vi "Complex Matrix Trace.vi"(0 "Input Matrix":T1) -> (1 "trace":cdb format="%.2f", 2 "error":i32)   [LabVIEW 2014, in "NI_AALPro.lvlib"]
doc: "Finds the <B>trace</B> of <B>Input Matrix</B>. Wire data to the <B>Input Matrix</B> input to determine the polymorphic instance to use or manually select the instance."
uses:
  NI_AALPro.lvlib
  ComplexMatrix.ctl
  lvanlys.dll
  NI_Matrix.lvlib
panel:
  # "Complex Matrix Trace"
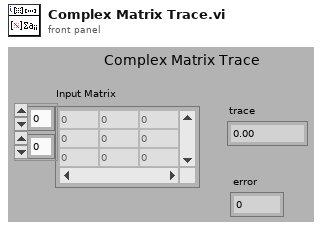
[diagram p1: front panel]
types:
  T1 = typedef "NI_Matrix.lvlib/ComplexMatrix.ctl" = cdb[][]
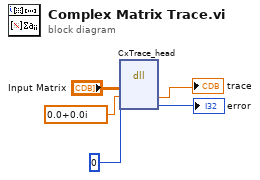
[diagram p0: block diagram]
diagram:
  n1 = dll-call lib="C:/Program Files (x86)/National Instruments/LabVIEW 2014/resource/lvanlys.*" fn="CxTrace_head"("Input Matrix"="Input Matrix", cdb 0.0+0.0i, 0) -> (→"trace":cdb, →"error":i32)  [unwired: 5 in, 2 out]
